vi "LUnit Stop Test.vi"(8 "error in (no error)":errorcluster, 11 "Coverage Report in":refnum<class "Coverage Report.lvclass">) -> (0 "error out":errorcluster, 3 "Coverage Report out":refnum<class "Coverage Report.lvclass">)   [LabVIEW 2020, in "Coverage Report.lvclass"]
uses:
  Coverage Report.lvclass
  Coverage Report.lvclass/Coverage Report.ctl
  <vilib>/Platform/browser.llb/Open URL in Default Browser (path).vi
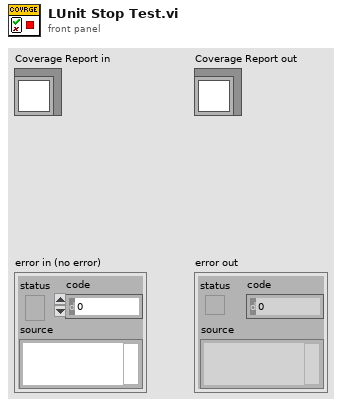
[diagram p1: front panel]
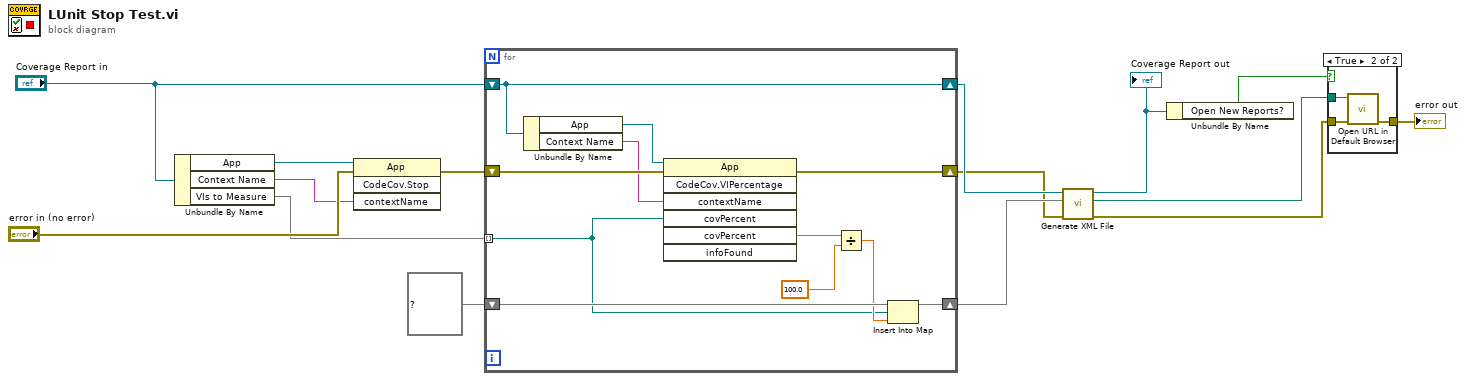
[diagram p0: block diagram]
diagram:
  n1 = Unbundle By Name("Coverage Report in") -> ("App"=w13:refnum<vi>, "Context Name"=w10:string, "VIs to Measure"=w2:set{path})
  n2 = invoke class="App" method="CodeCov.Stop"(reference=w13, error in="error in (no error)", "contextName"=w10) -> (error out=w1:errorcluster)  [unwired: 1 in, 3 out]
  n3 = for {
    shift-right: [w20] -> w9
    shift-left: "Coverage Report in" -> [w20]
    shift-right: [w25] -> w7
    shift-left: w1 -> [w26]
    shift-right: [w23] -> w8
    shift-left: map{path, dbl} {} ("Code Coverage") -> [w24]
    tunnel: w2 -> [w16] mode=indexing
    n4 = Unbundle By Name(w20) -> ("App"=w22:refnum<vi>, "Context Name"=w17:string)
    n5 = invoke class="App" method="CodeCov.VIPercentage"(reference=w22, error in=w26, "contextName"=w17, "covPercent"=w16) -> (error out=w25:errorcluster, "covPercent"=w21:dbl)  [unwired: 3 in, 5 out]
    n6 = Divide(x=w21, y=100.0) -> (x/y=w19:dbl)
    n7 = Insert Into Map(map in=w24, key=w16, value=w19) -> (map out=w23:map{path, dbl})  [unwired: 2 out]
  }
  n8 = call "Generate XML File.vi"("error in (no error)"=w7, "Code Coverage"=w8, "Coverage Report in"=w9) -> ("error out"=w6:errorcluster, "Report Path"=w3:path, "Coverage Report out"=w5:refnum<class "Coverage Report.lvclass">)  [unwired: 6 in]
  "Coverage Report out" <- w5
  n9 = Unbundle By Name(w5) -> ("Open New Reports?"=w4:bool)
  n10 = case shown="True" w4 {
    tunnel: w6 -> [w27 w30]
    tunnel: [w27 w29] -> w15
    tunnel: w3 -> [_ w28]
    frame False {
    }
    frame True {
      n11 = call-poly <vilib>:"Open URL in Default Browser.vi"("error in (no error)"=w30, "path"=w28) -> ("error out"=w29:errorcluster)  [unwired: 4 in, 1 out]
    }
  }
  "error out" <- w15
